vi "Main.vi"() -> ()   [LabVIEW 2023, in "Example Device.lvclass"]
uses:
  Example Device.lvclass
  Example Device.lvclass/Example Device.ctl
  Current Setpoint/Current Setpoint.lvclass
  D:/Labview/bls-capabilities-bto/Setpoint/Setpoint.lvclass
  Setpoint/Setpoint.lvclass
  Current Actual Value/Current Actual Value.lvclass
  Voltage Actual Value/Voltage Actual Value.lvclass
  D:/Labview/bls-capabilities-bto/Capabilities/Capabilities.lvclass
  D:/Labview/bls-capabilities-bto/Current Setpoint/Current Setpoint.lvclass
  Voltage Setpoint/Voltage Setpoint.lvclass
  D:/Labview/bls-capabilities-bto/Voltage Setpoint/Voltage Setpoint.lvclass
panel:
  in  "Voltage.AV":dbl[](array[numeric])
  in  "Current.AV":dbl[](array[numeric])
  out "Voltage.SP":dbl[](array[numeric])
  in  "stop":bool
  out "Current.SP":dbl[](array[numeric])
  in  "Number of Channels":u32=1
  in  "ExampleDevice.lvclass":refnum<class "Example Device.lvclass">
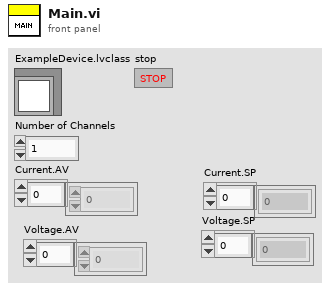
[diagram p1: front panel]
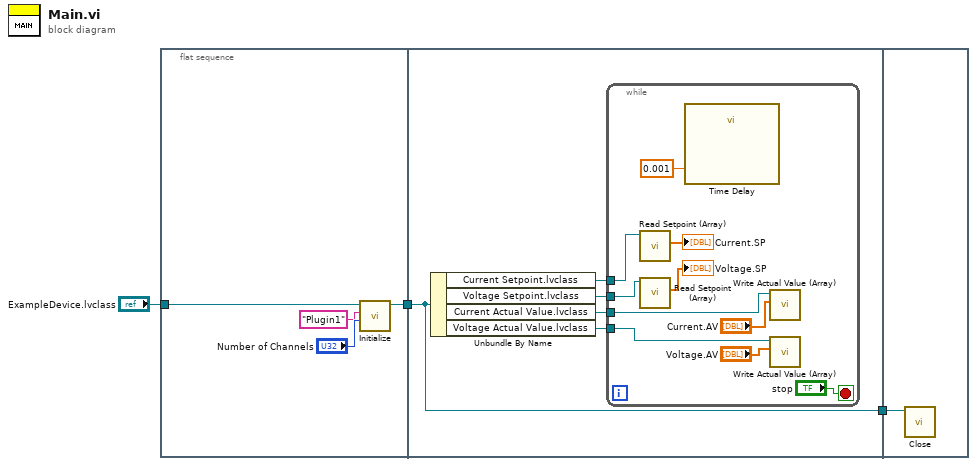
[diagram p0: block diagram]
diagram:
  n1 = flat-sequence {
    tunnel: "ExampleDevice.lvclass" -> [w7]
    tunnel: [w6] -> w2
    tunnel: w2 -> [w12]
    tunnel: [w12] -> w1
    tunnel: w1 -> [w23]
    frame #0 {
      n2 = call-dynamic "Initialize.vi"("Number of Channels"="Number of Channels", "Instance Name"="Plugin1" ("Plugin Name"), "ExampleDevice in"=w7) -> ("ExampleDevice out"=w6:refnum<class "Example Device.lvclass">)  [unwired: 7 in, 1 out]
    }
    frame #1 {
      n3 = Unbundle By Name(w12) -> ("Current Setpoint.lvclass"=w11:refnum<class "Current Setpoint.lvclass">, "Voltage Setpoint.lvclass"=w10:refnum<class "Voltage Setpoint.lvclass">, "Current Actual Value.lvclass"=w9:refnum<class "Current Actual Value.lvclass">, "Voltage Actual Value.lvclass"=w8:refnum<class "Voltage Actual Value.lvclass">)
      n4 = while {
        tunnel: w11 -> [w22]
        tunnel: w10 -> [w16]
        tunnel: w9 -> [w18]
        tunnel: w8 -> [w17]
        stop <- "stop" stop-if-true
        n5 = call "Read Setpoint (Array).vi"("Setpoint.lvclass"=w22) -> ("Current Setpoint"=→"Current.SP":dbl[])  [unwired: 7 in, 3 out]
        n6 = call "Read Setpoint (Array).vi"("Setpoint.lvclass"=w16) -> ("Current Setpoint"=→"Voltage.SP":dbl[])  [unwired: 7 in, 3 out]
        n7 = call "Time Delay"("Delay Time (s)"=0.001) -> ()  [unwired: 10 in, 1 out]
        n8 = call-dynamic "Write Actual Value (Array).vi"("Actual Value"="Current.AV", "Actual Value in"=w18) -> ()  [unwired: 8 in, 2 out]
        n9 = call-dynamic "Write Actual Value (Array).vi"("Actual Value"="Voltage.AV", "Actual Value in"=w17) -> ()  [unwired: 8 in, 2 out]
      }
    }
    frame #2 {
      n10 = call-dynamic "Close.vi"("ExampleDevice in"=w23) -> ()  [unwired: 9 in, 2 out]
    }
  }
